vi "Intake.Begin.vi"(8 "error in (no error)":errorcluster) -> (0 "error out":errorcluster)   [LabVIEW 2020]
doc: "Begin for Begin\n\nInput:\n -- error in -- cluster\n\nOutput:\n -- error out -- cluster"
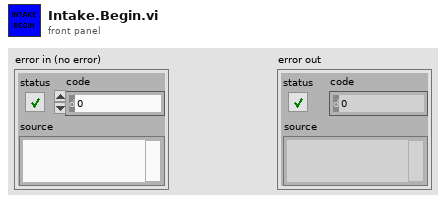
[diagram p1: front panel]
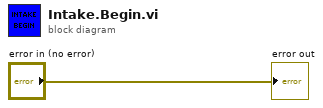
[diagram p0: block diagram]
diagram:
  "error out" <- "error in (no error)"
